vi "Write data to tdms file (PC VI).vi"() -> ()   [LabVIEW 2019]
uses:
  <resource>/objmgr/ni.dex.rc
panel:
  in  "base path (do not change)":path=path "D:/"
  in  "file name or relative path (e.g. \"something.tdms\")":string="Test.tdms"
  out "Available Elements for Reading":i32
  out "error out":errorcluster
  # "Start this script first"
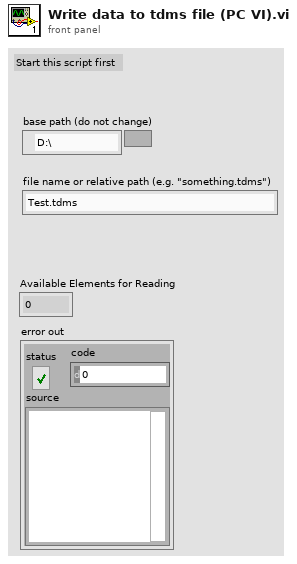
[diagram p1: front panel]
types:
  T1 = enum16{"open", "open or create", "create or replace", "create", "open (read-only)"}
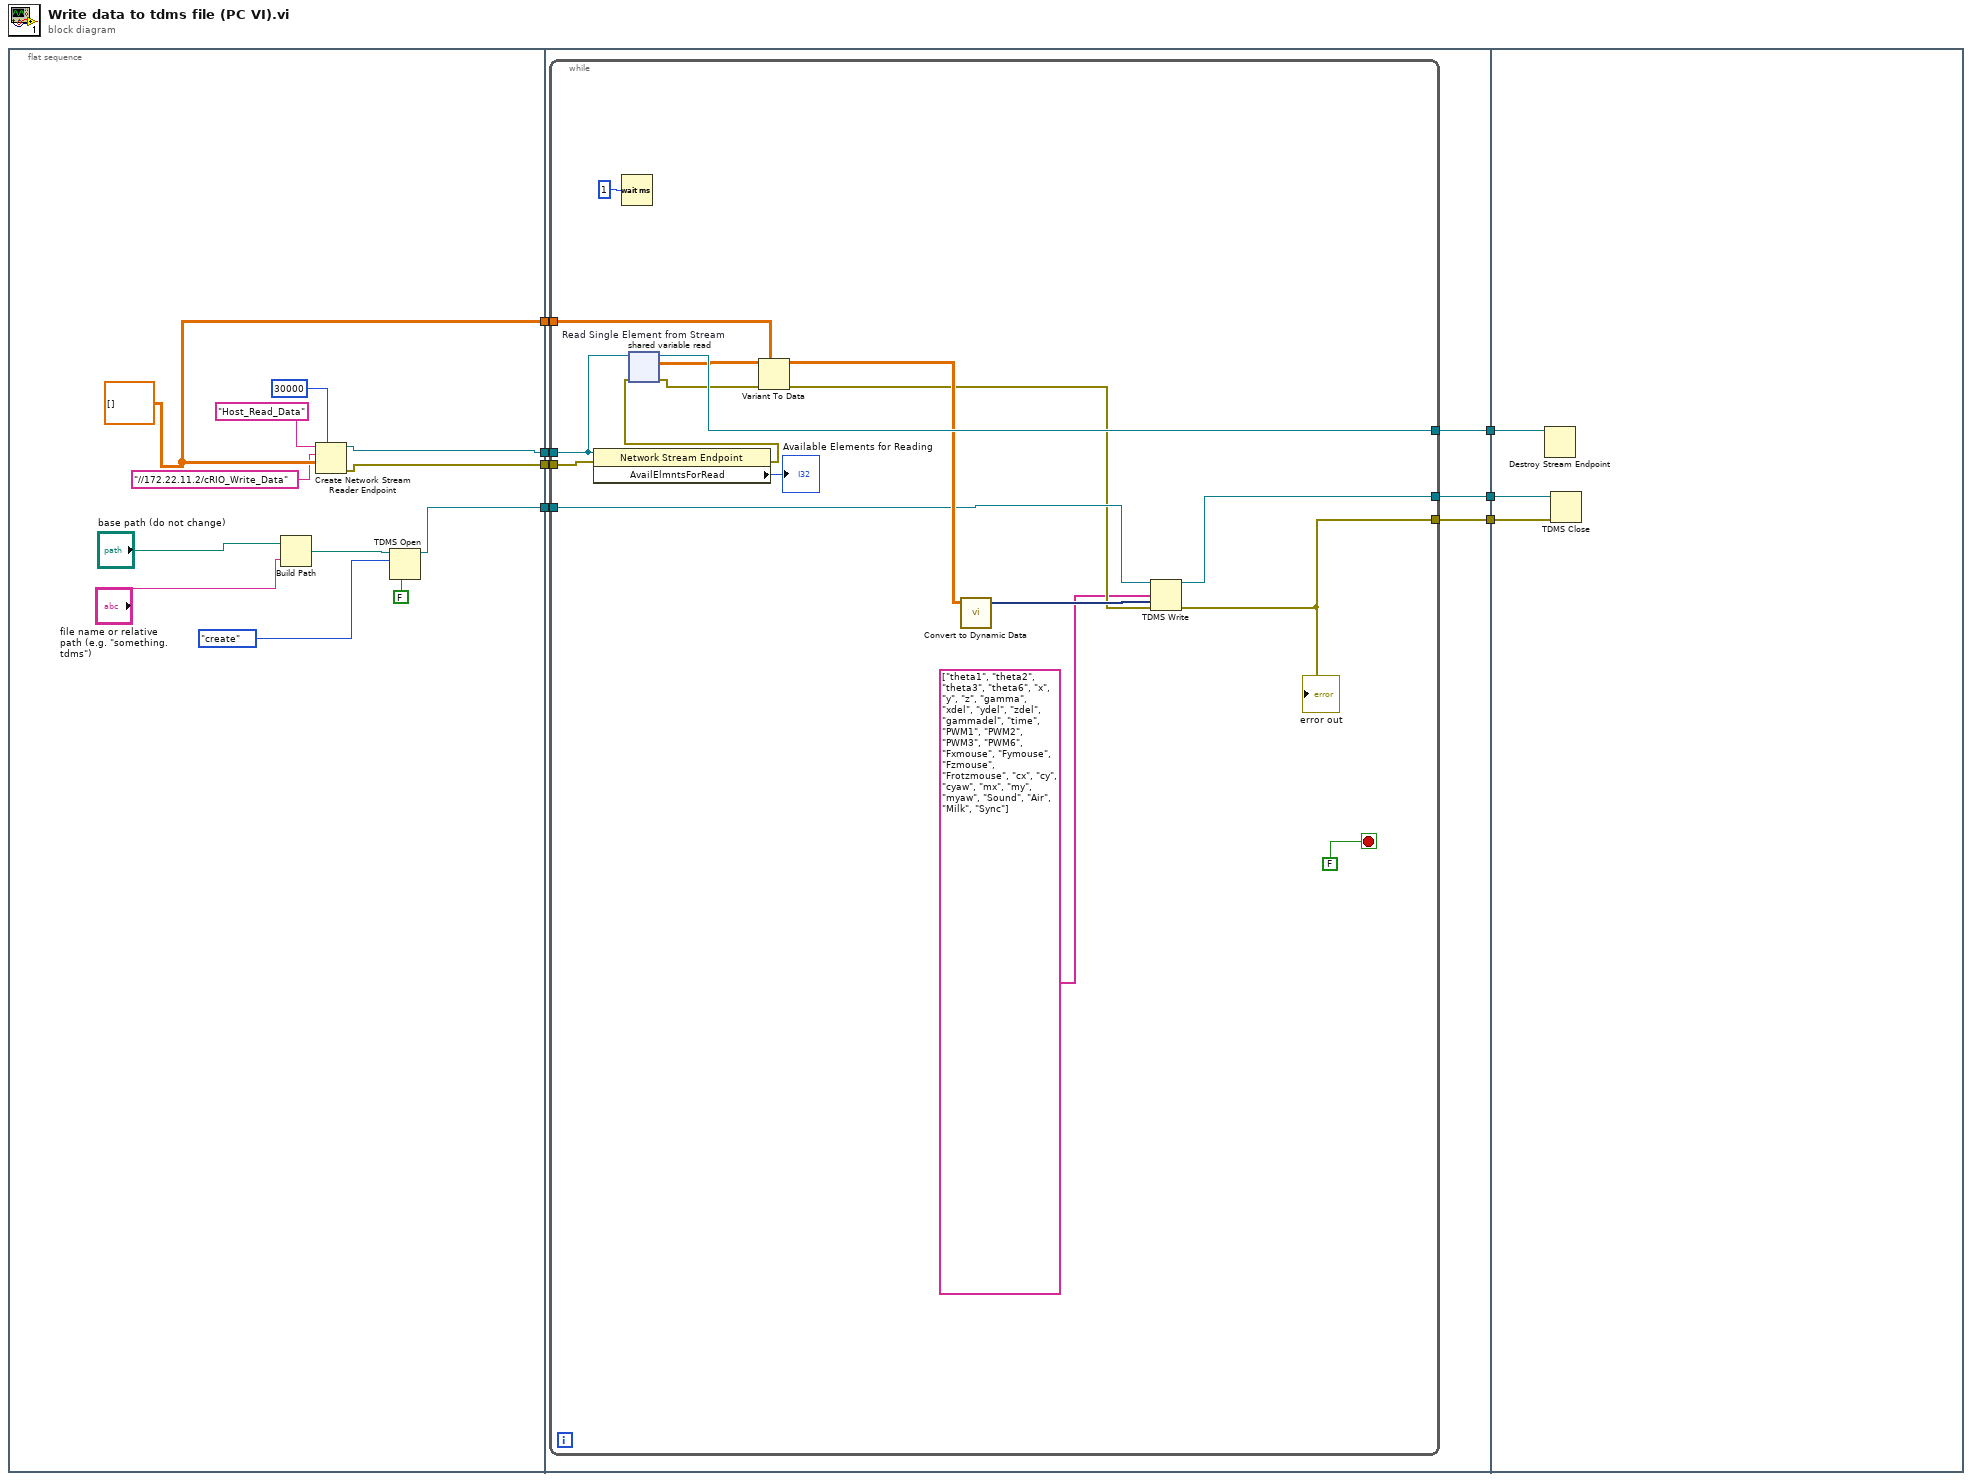
[diagram p0: block diagram]
diagram:
  n1 = flat-sequence {
    tunnel: [w11] -> w7
    tunnel: [w14] -> w6
    tunnel: [w13] -> w5
    tunnel: [w12] -> w1
    tunnel: w7 -> [w26]
    tunnel: [w25] -> w4
    tunnel: w6 -> [w24]
    tunnel: w5 -> [w23]
    tunnel: [w22] -> w3
    tunnel: [w21] -> w2
    tunnel: w1 -> [w20]
    tunnel: w4 -> [w46]
    tunnel: w3 -> [w45]
    tunnel: w2 -> [w44]
    frame #0 {
      w13 = dbl[][] [] ("array")
      n2 = Build Path(base path="base path (do not change)", name or relative path="file name or relative path (e.g. \"something.tdms\")") -> (appended path=w15:path)
      n3 = Create Network Stream Reader Endpoint(7:30000 ("reader buffer size"), 9:w13, 10:"//172.22.11.2/cRIO_Write_Data" ("writer url"), 11:"Host_Read_Data" ("reader name")) -> (0:w12:errorcluster, 3:w11:refnum<k21>)  [unwired: 3 in]
      n4 = TDMS Open(6:FALSE ("disable buffering (T)"), 10:T1."create" ("operation"), 11:w15) -> (3:w14:refnum<k34>)  [unwired: 4 in, 1 out]
    }
    frame #1 {
      n5 = while {
        tunnel: w26 -> [w40]
        tunnel: [w42] -> w25
        tunnel: w24 -> [w32]
        tunnel: w23 -> [w37]
        tunnel: [w31] -> w22
        tunnel: w20 -> [w34]
        tunnel: [w28] -> w21
        stop <- FALSE stop-if-true
        n6 = property class="Network Stream Endpoint"(reference=w40, error in=w34) -> (error out=w33:errorcluster, "AvailElmntsForRead"=→"Available Elements for Reading":i32)  [unwired: 1 out]
        n7 = Wait (ms)(milliseconds to wait=u32 1) -> ()  [unwired: 1 out]
        n8 = shared-variable-read "Read Single Element from Stream"(w40, w33) -> (w42:refnum<k21>, w36:errorcluster, w38:dbl[][])  [unwired: 1 in, 1 out]
        n9 = Variant To Data(error in=w36, type=w37, Variant=w38) -> (data=w35:dbl[][], error out=w29:errorcluster)
        n10 = call "Convert to Dynamic Data"("2D Array"=w35) -> ("Dynamic Data Type"=w30:dynamicdata)  [unwired: 3 in]
        n11 = TDMS Write(0:w32, 7:string[] ["theta1", "theta2", "theta3", "theta6", "x", "y", "z", "gamma", "xdel", "ydel", "zdel", "gammadel", "time", "PWM1", "PWM2", "PWM3", "PWM6", "Fxmouse", "Fymouse", "Fzmouse", "Frotzmouse", "cx", "cy", "cyaw", "mx", "my", "myaw", "Sound", "Air", "Milk", "Sync"] ("channel name(s) in (Untitled)"), 9:w30, 11:w29) -> (4:w31:refnum<k34>, 15:w28:errorcluster)  [unwired: 2 in, 2 out]
        "error out" <- w28
      }
    }
    frame #2 {
      n12 = Destroy Stream Endpoint(11:w46) -> ()  [unwired: 1 in, 1 out]
      n13 = TDMS Close(8:w44, 11:w45) -> ()  [unwired: 2 out]
    }
  }
